vi "Launch Nested Views.vi"(8 "error in (no error)":errorcluster, 9 "View Labels (optional)":string[](array[string]), 10 "Viewables":refnum<class "IViewable.lvclass">[](array[class]), 11 "IViewManager In":refnum<class "IViewManager.lvclass">) -> (0 "error out":errorcluster, 3 "IViewManager Out":refnum<class "IViewManager.lvclass">)   [LabVIEW 2017, in "IViewManager.lvlib" / "IViewManager.lvclass"]
doc: "<License>\nCopyright © 2017 Composed Systems, LLC | All rights reserved\nwww.composed.io\n\nAuthor: Ethan Stern <ethan.stern@composed.io>\n\nThis software is provided \"AS IS\" WITHOUT WARRANTIES, either express or implied, AND IS FOR EDUCATIONAL PURPOSES ONLY.\n</License>"
uses:
  IViewManager.lvclass
  C:/Program Files (x86)/National Instruments/LabVIEW 2017/vi.lib/ActorFramework/Actor/Actor.lvclass
  C:/Git/mva-framework/Source/Framework/IViewable/IViewable/IViewable.lvclass
  IViewable/IViewable/IViewable.lvclass
  C:/Git/mva-framework/Source/Framework/IObserver/IObserver/IObserver.lvclass
  IViewable/IViewable/IViewable.lvclass/IViewable.ctl
  IObserver/IObserver/IObserver.lvclass/IObserver.ctl
  IViewable/IViewable/Write Application Style Reference.vi
  IViewable/IViewable/Read Application Style Reference.vi
  IObserver/IObserver/Transfer Observer Resources.vi
  <vilib>/ActorFramework/Actor/Actor.lvclass
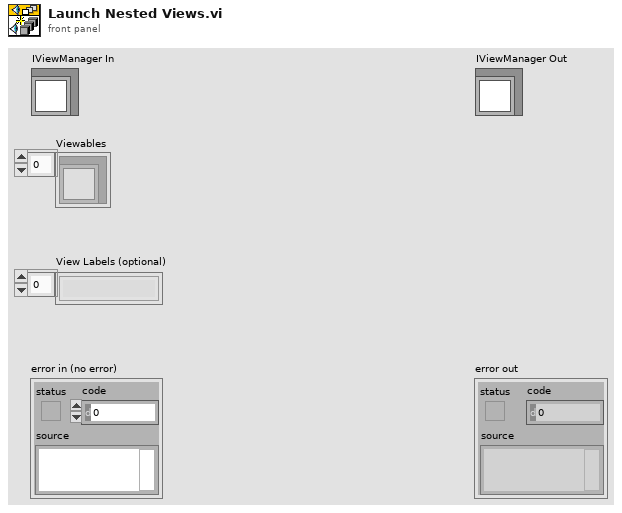
[diagram p1: front panel]
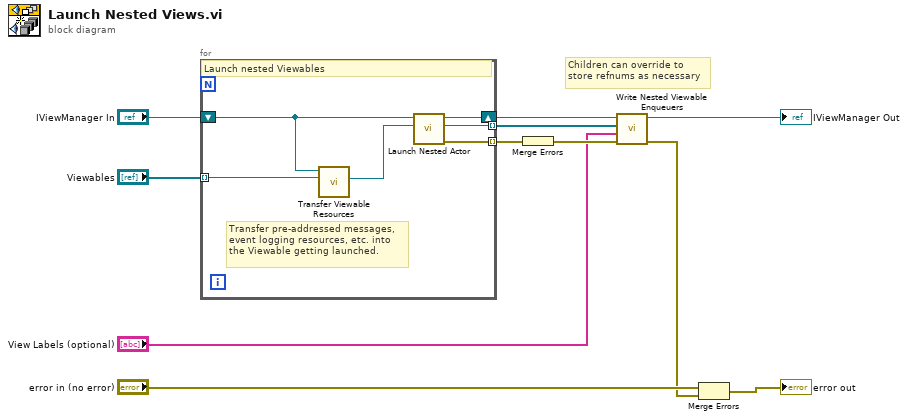
[diagram p0: block diagram]
diagram:
  # "Children can override to\nstore refnums as necessary"
  n1 = for {
    shift-right: [w17] -> w7
    shift-left: "IViewManager In" -> [w13]
    tunnel: "Viewables" -> [w16] mode=indexing
    tunnel: [w15] -> w4 mode=indexing
    tunnel: [w14] -> w8 mode=indexing
    # "Transfer pre-addressed messages,\nevent logging resources, etc. into\nthe Viewable getting launched."
    # "Launch nested Viewables"
    n2 = call "Transfer Viewable Resources.vi"("Recipient Viewable In"=w16, "Running Viewable"=w13) -> ("Recipient Viewable Out"=w12:refnum<class "IViewable.lvclass">)  [unwired: 9 in]
    n3 = call <vilib>:"Launch Nested Actor.vi"("Nested Actor"=w12, "Caller Actor in"=w13) -> ("error out"=w14:errorcluster, "Nested Actor's Enqueuer"=w15:refnum<class "Message Enqueuer.lvclass">, "Caller Actor out"=w17:refnum<class "IViewManager.lvclass">)  [unwired: 7 in]
  }
  n4 = Merge Errors(w8) -> (w5:errorcluster)
  n5 = call-dynamic "Write Nested Viewable Enqueuers.vi"("error in (no error)"=w5, "Viewable Names (optional)"="View Labels (optional)", "Nested Viewable Enqueuers"=w4, "IViewManager In"=w7) -> ("error out"=w3:errorcluster, "IViewManager Out"=→"IViewManager Out":refnum<class "IViewManager.lvclass">)  [unwired: 6 in]
  n6 = Merge Errors("error in (no error)", w3) -> (→"error out":errorcluster)
